vi "SeCrTs-DO_Write.vi"(7 "Data FIFO Ref":T1, 8 "error in (no error)":errorcluster, 11 "Refnum in":refnum<k21>) -> (0 "error out":errorcluster, 3 "Refnum out":refnum<k21>)   [LabVIEW 2022 SP3]
uses:
  RT Controls/SeCrTs-Data FIFO.ctl
  <vilib>/Platform/TimedLoop/XDataNode/timing_clust.ctl
  <vilib>/Platform/TimedLoop/XDataNode/nitl_modes.ctl
  <vilib>/Platform/TimedLoop/XDataNode/wakeup.ctl
  <vilib>/DAQmx/write.llb/DAQmx Write (Digital 1D Bool NChan 1Samp 1Line).vi
  <vilib>/DAQmx/miscellaneous.llb/DAQmx Fill In Error Info.vi
  <vilib>/platform/TimedLoop/XDataNode/XDataNode.xnode
  <vilib>/Platform/TimedLoop/XDataNode/XDNodeRunTimeDep.lvlib
panel:
  out "All data out":waveform(dbl)[](array[waveform])
  out "overflow?":bool
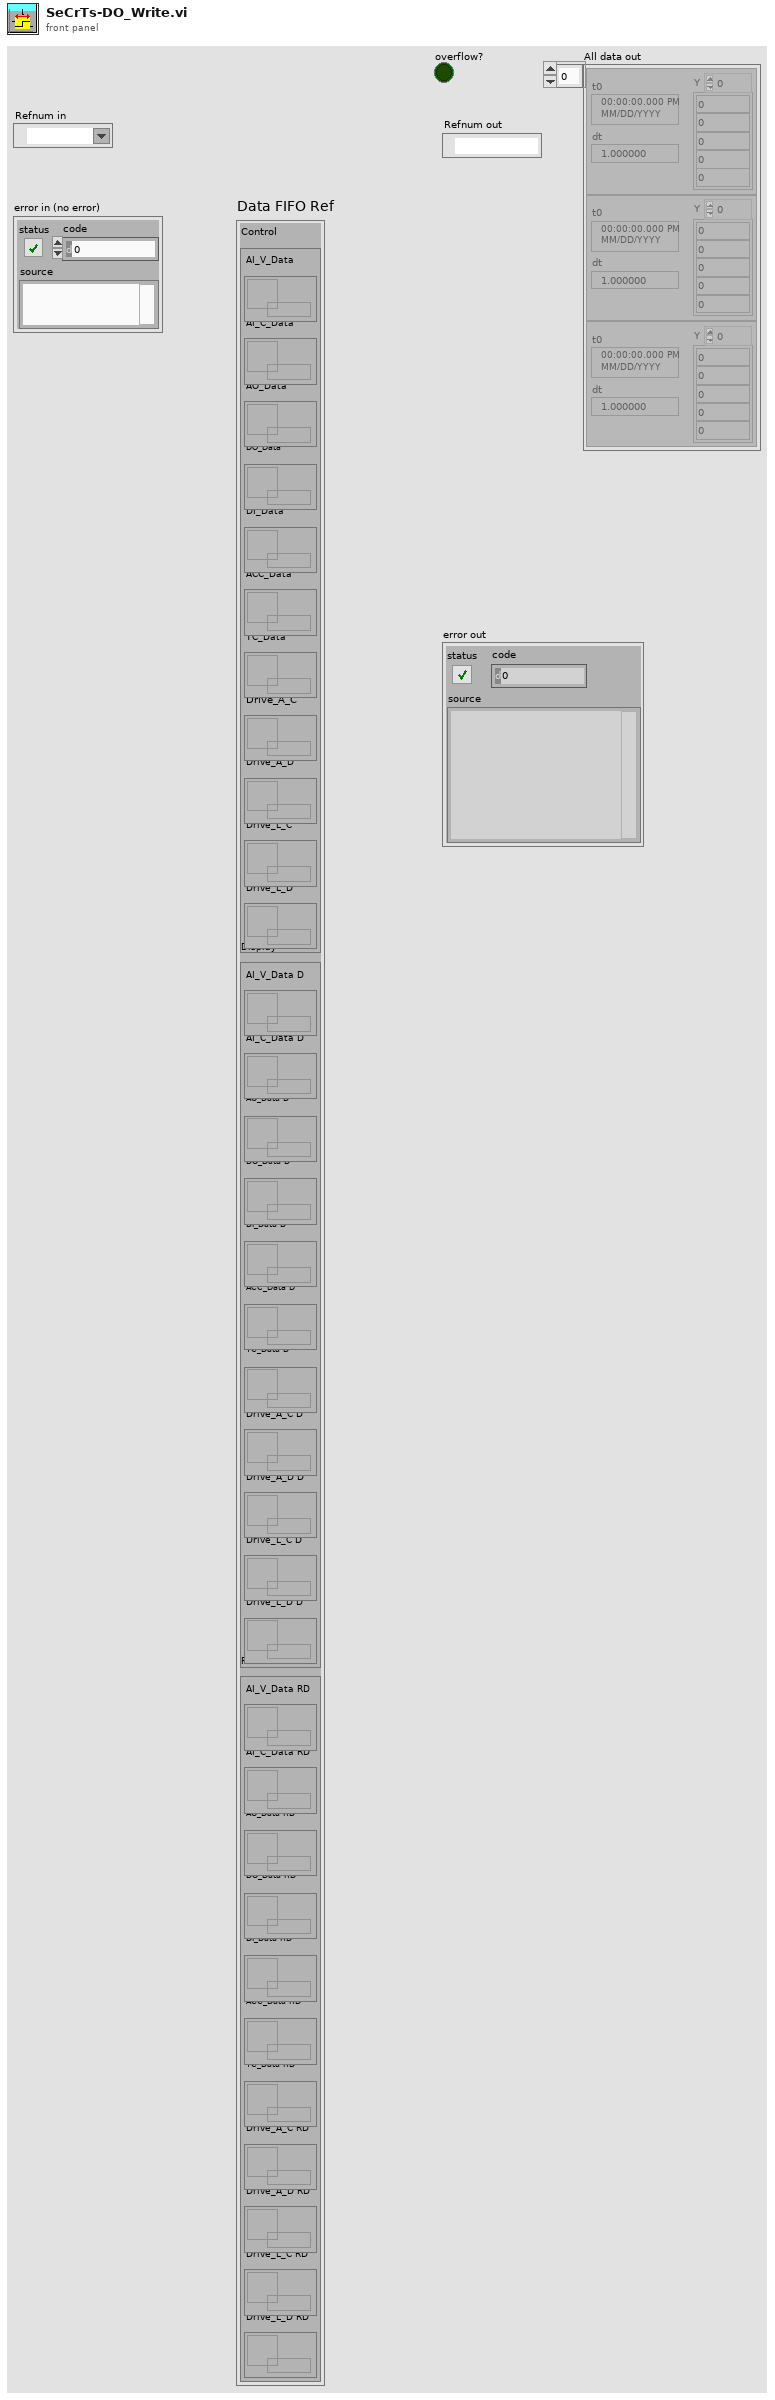
[diagram p1: front panel]
types:
  T1 = typedef "SeCrTs-Data FIFO.ctl" = cluster{"Control":cluster{"AI_V_Data":refnum<queue>, "AI_C_Data":refnum<queue>, "AO_Data":refnum<queue>, "DO_Data":refnum<queue>, "DI_Data":refnum<queue>, "ACC_Data":refnum<queue>, "TC_Data":refnum<queue>, "Drive_A_C":refnum<queue>, "Drive_A_D":refnum<queue>, "Drive_L_C":refnum<queue>, "Drive_L_D":refnum<queue>}, "Display":cluster{"AI_V_Data D":refnum<queue>, "AI_C_Data D":refnum<queue>, "AO_Data D":refnum<queue>, "DO_Data D":refnum<queue>, "DI_Data D":refnum<queue>, "ACC_Data D":refnum<queue>, "TC_Data D":refnum<queue>, "Drive_A_C D":refnum<queue>, "Drive_A_D D":refnum<queue>, "Drive_L_C D":refnum<queue>, "Drive_L_D D":refnum<queue>}, "RD":cluster{"AI_V_Data RD":refnum<queue>, "AI_C_Data RD":refnum<queue>, "AO_Data RD":refnum<queue>, "DO_Data RD":refnum<queue>, "DI_Data RD":refnum<queue>, "ACC_Data RD":refnum<queue>, "TC_Data RD":refnum<queue>, "Drive_A_C RD":refnum<queue>, "Drive_A_D RD":refnum<queue>, "Drive_L_C RD":refnum<queue>, "Drive_L_D RD":refnum<queue>}}
  T2 = typedef "XDNodeRunTimeDep.lvlib/timing_clust.ctl" = cluster{"Expected End [f-1]":u64, "Actual End [f-1]":u64, "Finished Late? [f-1]":bool, "Expected End [i-1]":u64, "Actual End [i-1]":u64, "Finished Late? [i-1]":bool, "Expected Start [i]":u64, "Actual Start [i]":u64, "Expected Start [f]":u64, "Actual Start [f]":u64, "Source Name":string, "Structure Name":string, "Period":i64, "Deadline":i64, "Offset":i64, "Start":i64, "Priority":i32, "Timeout":i32, "Mode":T3, "Wakeup Reason":T4, "Error":errorcluster, "Source Type":string, "Secondary Source Type":string, "Global End Time":u64, "Global Start Time":u64, "Frame Duration":u64, "Iteration Duration":u64, "Assigned CPU":i32, "I/O Scan Engine Mode":u32}
  T3 = typedef "XDNodeRunTimeDep.lvlib/nitl_modes.ctl" = enum32{"No Change", "Process missed periods, maintain original phase", "Discard missed periods, maintain original phase", "Process missed periods, ignore original phase", "Discard missed periods, ignore original phase"}
  T4 = typedef "XDNodeRunTimeDep.lvlib/wakeup.ctl" = enum32{"Normal", "Aborted", "Asynchronous wakeup", "Timing source error", "Timed loop error", "Timeout"}
  T5 = enum16{"Init", "Read", "Write 'All'", "Write 'n'", "Write Safe Value", "Write Start Time", "Overwrite Pattern", "Overwrite Pattern with Start", "Append Pattern", "Start Pattern Mode", "Abort Pattern Mode", "Read 1"}
  T6 = enum16{"AI C", "AI V", "AO", "DI", "DO", "TC", "ACC", "DR L", "DR A"}
  T7 = enum16{"Init", "Read 'All'", "Read 'n'", "Read '1'", "Write '1'", "Write 'n'", "Write 'All'"}
  T8 = cluster{"Start DAQ":bool, "Stop DAQ":bool, "RT Stop":bool, "RT Exit":bool, "Start Seq":bool}
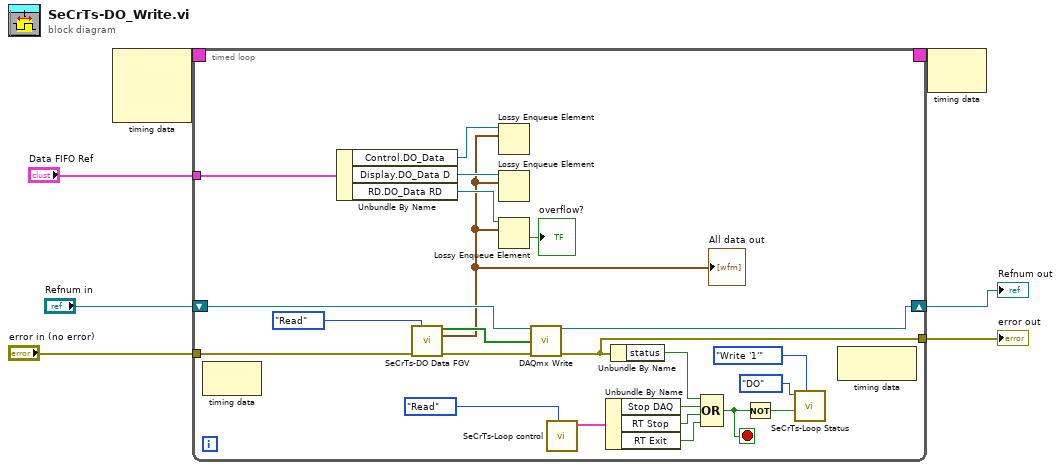
[diagram p0: block diagram]
diagram:
  n1 = node-c288() -> (w7:T2)  [unwired: 3 in]
  n2 = timed-loop {
    tunnel: "error in (no error)" -> [w12]
    tunnel: [w29] -> w4
    timing: w7 -> [_]
    timing-out: [_] -> w6
    tunnel: "Data FIFO Ref" -> [w21]
    shift-right: [w9] -> w1
    shift-left: "Refnum in" -> [w28]
    stop <- w30 stop-if-true
    n3 = node-c288() -> ()  [unwired: 1 in, 1 out]
    n4 = Unbundle By Name(w21) -> ("Control.DO_Data"=w20:refnum<queue>, "Display.DO_Data D"=w19:refnum<queue>, "RD.DO_Data RD"=w18:refnum<queue>)
    n5 = call "SeCrTs-DO Data FGV.vi"("Option"=T5."Read", "error in (no error)"=w12) -> ("DO Values Out"=w13:bool[], "All data out"=w10:waveform(dbl)[], "error out"=w11:errorcluster)  [unwired: 7 in, 4 out]
    "All data out" <- w10
    n6 = Lossy Enqueue Element(queue=w20, element=w10) -> ()  [unwired: 1 in, 4 out]
    n7 = Lossy Enqueue Element(queue=w19, element=w10) -> ()  [unwired: 1 in, 4 out]
    n8 = Lossy Enqueue Element(queue=w18, element=w10) -> (overflow?=→"overflow?":bool)  [unwired: 1 in, 3 out]
    n9 = call-poly <vilib>:"DAQmx Write.vi"("task/channels in"=w28, "data"=w13, "error in"=w11) -> ("task out"=w9:refnum<k21>, "error out"=w29:errorcluster)  [unwired: 10 in, 1 out]
    n10 = call "SeCrTs-Loop control.vi"("Action"=enum16{"Init", "Write", "Read"}."Read") -> ("Loop Control out"=w26:T8)  [unwired: 9 in, 1 out]
    n11 = Unbundle By Name(w26) -> ("Stop DAQ"=w25:bool, "RT Stop"=w24:bool, "RT Exit"=w23:bool)
    n12 = Unbundle By Name(w29) -> ("status"=w27:bool)
    n13 = Compound Arithmetic op=OR(w27, w25, w24, w23) -> (w30:bool)
    n14 = Not(x=w30) -> (.not. x?=w16:bool)
    n15 = call "SeCrTs-Loop Status.vi"("Option"=T7."Write '1'", "Status"=w16, "Loop"=T6."DO") -> ()  [unwired: 6 in, 3 out]
    n16 = node-c288() -> ()  [unwired: 1 in, 1 out]
  }
  "Refnum out" <- w1
  "error out" <- w4
  n17 = node-c288(w6) -> ()  [unwired: 1 out]
